vi "Create New Tags and Mappings.vi"(8 "write reservations in":cluster{"Array":T1[]}[](array[cluster]), 9 "read reservations in":cluster{"Array":T1[]}[](array[cluster]), 10 "module mapping":T2[](array[typedef]), 11 "main data dictionary in":refnum<class "data dictionary.lvclass">) -> (2 "module mapping":T2[](array[typedef]), 3 "main data dictionary out":refnum<class "data dictionary.lvclass">)   [LabVIEW 2013, in "Engine Runtime Interface.lvclass"]
uses:
  Engine Runtime Interface.lvclass
  Engine Configuration/Module Mappings.ctl
  <vilib>/NI/Tag Bus/table/mapping specification.ctl
  <vilib>/NI/Tag Bus/tag/Data Type.ctl
  <vilib>/NI/Tag Bus/table/mapping.ctl
  <vilib>/NI/Tag Bus/dictionary/data dictionary.lvclass
  <vilib>/NI/Tag Bus Module Framework/module configuration/channel reservation.ctl
  <vilib>/NI/Tag Bus Module Framework/channel/TBM channel.lvclass
  <vilib>/NI/Tag Bus/tag/tag descriptor.lvclass
  Engine Configuration/engine configuration.lvclass
  <vilib>/NI/Tag Bus/table/data table.lvlib
  <vilib>/NI/Tag Bus Module Framework/module configuration/TBM module configuration.lvclass
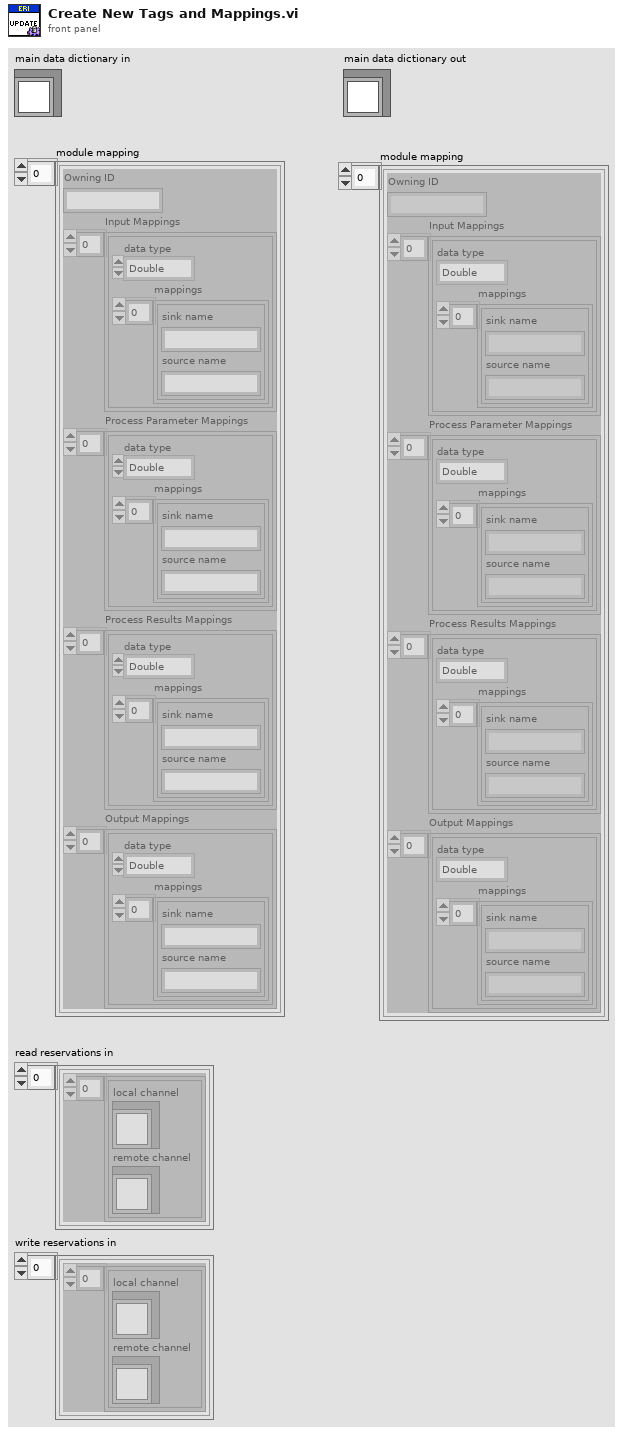
[diagram p1: front panel]
types:
  T1 = typedef "TBM module configuration.lvclass/channel reservation.ctl" = cluster{"local channel":refnum<class "TBM channel.lvclass">, "remote channel":refnum<class "TBM channel.lvclass">}
  T2 = typedef "engine configuration.lvclass/Module Mappings.ctl" = cluster{"Owning ID":string, "Input Mappings":T3[], "Process Parameter Mappings":T3[], "Process Results Mappings":T3[], "Output Mappings":T3[]}
  T3 = typedef "tag bus.lvlib/data table.lvlib/mapping specification.ctl" = cluster{"data type":T4, "mappings":T5[]}
  T4 = typedef "tag bus.lvlib/tag descriptor.lvclass/Data Type.ctl" = enum16{"Double", "Single", "I64", "I32", "I16", "I8", "U64", "U32", "U16", "U8", "Boolean", "String", "Array of Double", "Array of Single", "Array of I64", "Array of I32", "Array of I16", "Array of I8", "Array of U64", "Array of U32", "Array of U16", "Array of U8", "Array of Boolean", "Array of String"}
  T5 = typedef "tag bus.lvlib/data table.lvlib/mapping.ctl" = cluster{"sink name":string, "source name":string}
  T6 = cluster{"Tag Name":string, "Channel Name":string}
  T7 = cluster{"Tag Name":string, "Channel Name":string}[]
  T8 = typedef "engine configuration.lvclass/Mappings.ctl" = cluster{"Data Type":T4, "Mappings":cluster{"Tag Name":string, "Channel Name":string}[]}
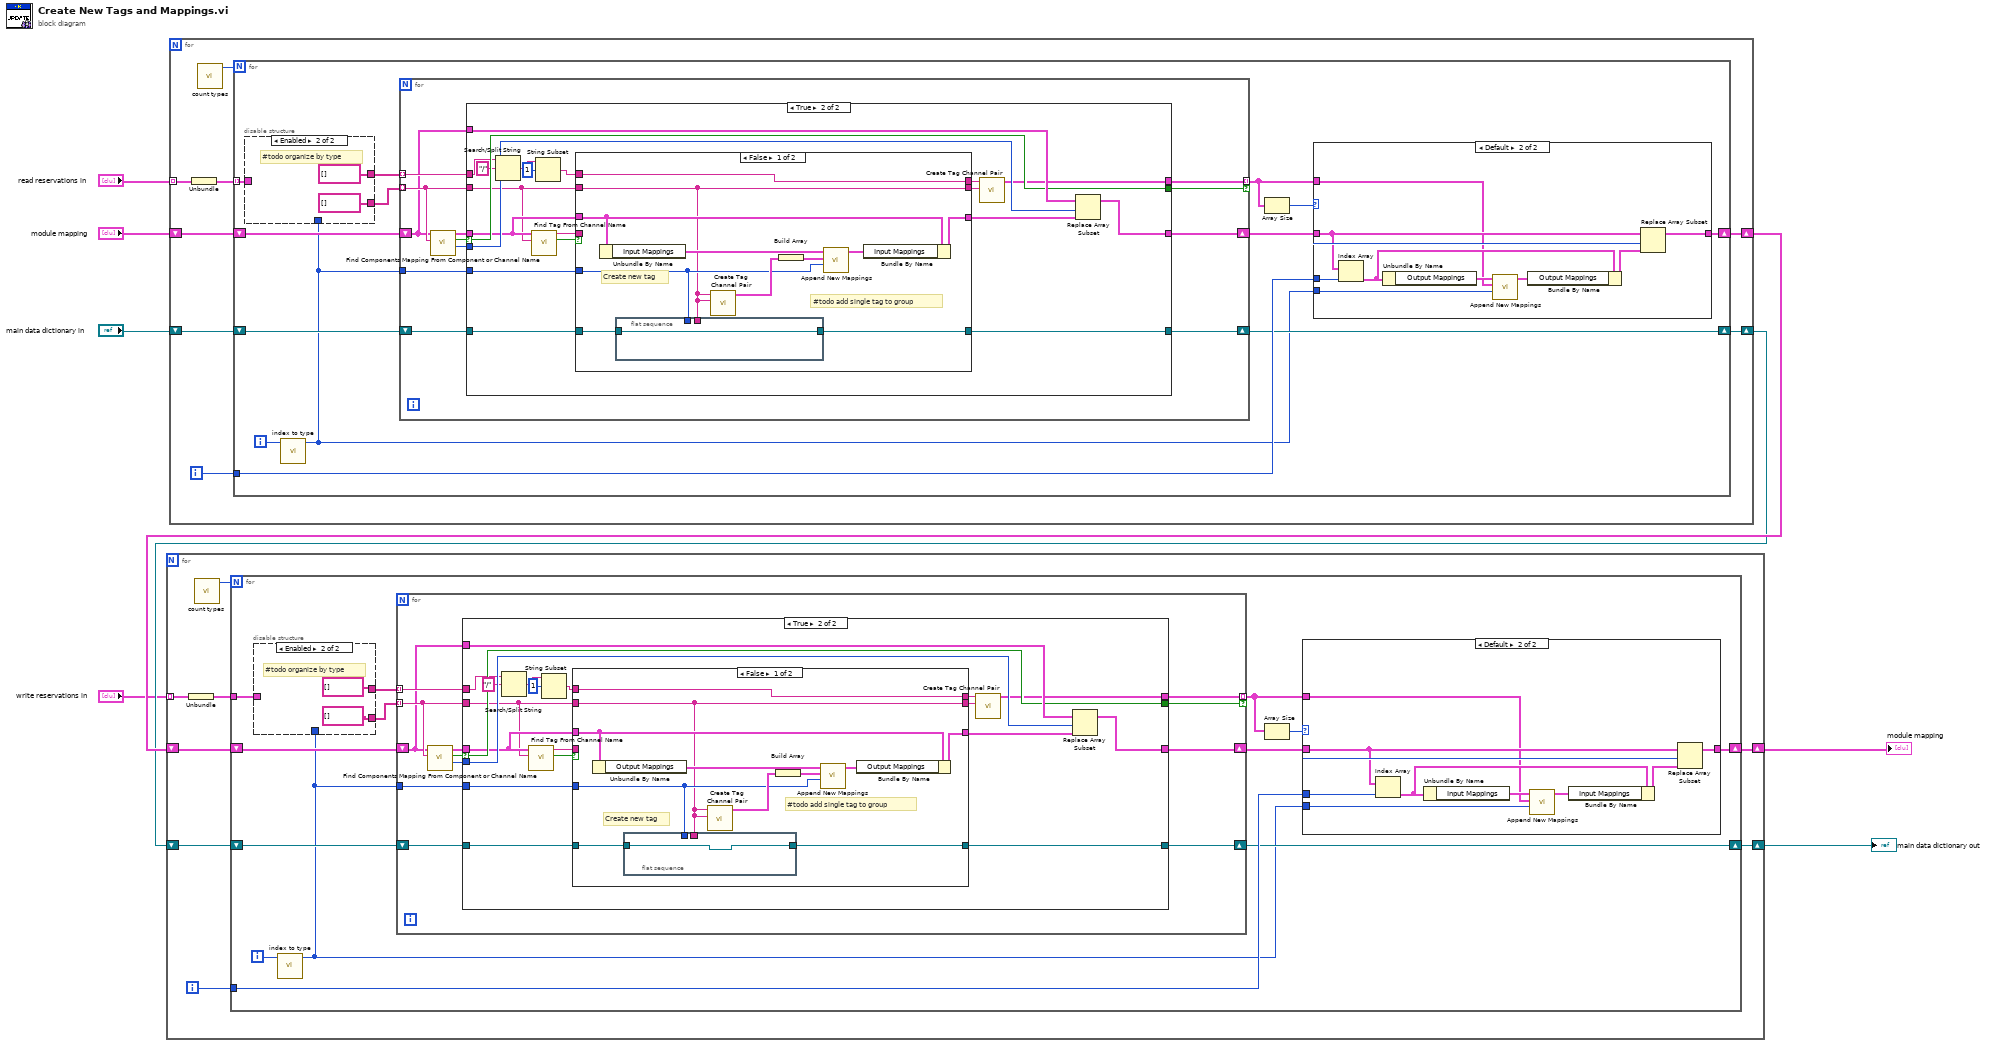
[diagram p0: block diagram]
diagram:
  n1 = for {
    tunnel: "read reservations in" -> [w16] mode=indexing
    shift-right: [w15] -> w6
    shift-left: "module mapping" -> [w12]
    shift-right: [w13] -> w5
    shift-left: "main data dictionary in" -> [w11]
    i -> [w14]
    n2 = Unbundle(w16) -> ("Array"=w9:T1[])
    n3 = call <vilib>:"count types.vi"() -> ("type count"=w10:i32)  [unwired: 11 in]
    n4 = for {
      N: w10 -> [_]
      tunnel: w9 -> [w22] mode=indexing
      tunnel: w14 -> [w28]
      shift-right: [w29] -> w15
      shift-left: w12 -> [w26]
      shift-right: [w27] -> w13
      shift-left: w11 -> [w25]
      i -> [w24]
      n5 = call <vilib>:"index to type.vi"("I32"=w24) -> ("type"=w19:T4)  [unwired: 10 in]
      n6 = disable-structure shown="Enabled" {
        disable-tunnel: w22 -> [_ _]
        disable-tunnel: [_ string[] [] ("tags")] -> w21
        disable-tunnel: [_ string[] [] ("tags")] -> w20
        disable-tunnel: w19 -> [_ _]
        frame Disabled {
        }
        frame Enabled {
          # "#todo organize by type"
        }
      }
      n7 = for {
        tunnel: w20 -> [w53] mode=indexing
        tunnel: [w52] -> w18 mode=indexing if=w44
        tunnel: w21 -> [w50] mode=indexing
        shift-right: [w46] -> w23
        shift-left: w26 -> [w47]
        shift-right: [w43] -> w27
        shift-left: w25 -> [w51]
        tunnel: w19 -> [w42]
        n8 = call "Find Components Mapping From Component or Channel Name.vi"("module/channel name"=w50, "module mapping"=w47) -> ("index"=w48:i32, "found?"=w45:bool, "found mapping"=w49:T2)  [unwired: 7 in]
        n9 = case shown="True" w45 {
          selector: w45 -> [w55 w71]
          tunnel: w53 -> [_ w61]
          tunnel: [_ w65] -> w52
          tunnel: w51 -> [w54 w76]
          tunnel: w50 -> [_ w68]
          tunnel: w49 -> [_ w69]
          tunnel: w48 -> [_ w74]
          tunnel: w47 -> [w56 w73]
          tunnel: [w56 w72] -> w46
          tunnel: [w55 w71] -> w44
          tunnel: [w54 w70] -> w43
          tunnel: w42 -> [_ w62]
          frame False {
          }
          frame True {
            n10 = Search/Split String(string=w61, search string/char (-)="/") -> (match + rest of string=w59:string)  [unwired: 1 in, 2 out]
            n11 = call "Find Tag From Channel Name.vi"("channel name"=w68, "Module Mappings"=w69) -> ("found?"=w67:bool, "mapped tag"=w66:string)  [unwired: 8 in]
            n12 = String Subset(string=w59, offset (0)=1) -> (substring=w57:string)  [unwired: 1 in]
            n13 = case shown="False" w67 {
              tunnel: w57 -> [w81 w90]
              tunnel: w66 -> [_ w89]
              tunnel: w68 -> [w77 _]
              tunnel: w76 -> [w80 w91]
              tunnel: w69 -> [w87 w92]
              tunnel: [w86 w92] -> w75
              tunnel: [w79 w91] -> w70
              tunnel: [w81 w90] -> w64
              tunnel: [w77 w89] -> w63
              tunnel: w62 -> [w78 _]
              frame False {
                # "#todo add single tag to group"
                # "Create new tag"
                n14 = Unbundle By Name(w87) -> ("Input Mappings"=w85:T3[])
                n15 = flat-sequence {
                  tunnel: w80 -> [w88]
                  tunnel: [w88] -> w79
                  tunnel: w78 -> [_]
                  tunnel: w77 -> [_]
                  frame #0 {
                  }
                }
                n16 = call "Create Tag Channel Pair.vi"("Tag Name"=w77, "Channel Name"=w77) -> ("tag channel pair"=w83:T6)  [unwired: 9 in]
                n17 = Build Array(w83) -> (w82:T7)
                n18 = call "Append New Mappings.vi"("Type"=w78, "Mappings to Append"=w82, "Mappings in"=w85) -> ("Mappings out"=w84:T8[])  [unwired: 8 in]
                n19 = Bundle By Name(cluster=w87, "Input Mappings"=w84) -> (w86:T2)
              }
              frame True {
              }
            }
            n20 = call "Create Tag Channel Pair.vi"("Tag Name"=w63, "Channel Name"=w64) -> ("tag channel pair"=w65:T6)  [unwired: 9 in]
            n21 = Replace Array Subset(array=w73, new element=w75, index=w74) -> (w72:T2[])
          }
        }
      }
      n22 = Array Size(array=w18) -> (size(s)=w17:i32)
      n23 = case shown="Default" w17 {
        tunnel: [w32 w41] -> w29
        tunnel: w28 -> [_ w40]
        tunnel: w23 -> [w32 w36]
        tunnel: w19 -> [_ w34]
        tunnel: w18 -> [_ w33]
        frame 0 {
        }
        frame Default {
          n24 = Index Array(array=w36, index=w40) -> (element=w39:T2)
          n25 = Unbundle By Name(w39) -> ("Output Mappings"=w35:T3[])
          n26 = call "Append New Mappings.vi"("Type"=w34, "Mappings to Append"=w33, "Mappings in"=w35) -> ("Mappings out"=w38:T8[])  [unwired: 8 in]
          n27 = Bundle By Name(cluster=w39, "Output Mappings"=w38) -> (w37:T2)
          n28 = Replace Array Subset(array=w36, new element=w37, index=w40) -> (w41:T2[])
        }
      }
    }
  }
  n29 = for {
    tunnel: "write reservations in" -> [w100] mode=indexing
    shift-right: [w99] -> w7
    shift-left: w6 -> [w96]
    shift-right: [w97] -> w3
    shift-left: w5 -> [w95]
    i -> [w98]
    n30 = Unbundle(w100) -> ("Array"=w93:T1[])
    n31 = call <vilib>:"count types.vi"() -> ("type count"=w94:i32)  [unwired: 11 in]
    n32 = for {
      N: w94 -> [_]
      tunnel: w93 -> [w106]
      tunnel: w98 -> [w112]
      shift-right: [w113] -> w99
      shift-left: w96 -> [w110]
      shift-right: [w111] -> w97
      shift-left: w95 -> [w109]
      i -> [w108]
      n33 = call <vilib>:"index to type.vi"("I32"=w108) -> ("type"=w103:T4)  [unwired: 10 in]
      n34 = disable-structure shown="Enabled" {
        disable-tunnel: w106 -> [_ _]
        disable-tunnel: [_ string[] [] ("tags")] -> w105
        disable-tunnel: [_ string[] [] ("tags")] -> w104
        disable-tunnel: w103 -> [_ _]
        frame Disabled {
        }
        frame Enabled {
          # "#todo organize by type"
        }
      }
      n35 = for {
        tunnel: w104 -> [w137] mode=indexing
        tunnel: [w136] -> w102 mode=indexing if=w128
        tunnel: w105 -> [w134] mode=indexing
        shift-right: [w130] -> w107
        shift-left: w110 -> [w131]
        shift-right: [w127] -> w111
        shift-left: w109 -> [w135]
        tunnel: w103 -> [w126]
        n36 = call "Find Components Mapping From Component or Channel Name.vi"("module/channel name"=w134, "module mapping"=w131) -> ("index"=w132:i32, "found?"=w129:bool, "found mapping"=w133:T2)  [unwired: 7 in]
        n37 = case shown="True" w129 {
          selector: w129 -> [w139 w155]
          tunnel: w137 -> [_ w142]
          tunnel: [_ w149] -> w136
          tunnel: w135 -> [w138 w160]
          tunnel: w134 -> [_ w152]
          tunnel: w133 -> [_ w153]
          tunnel: w132 -> [_ w158]
          tunnel: w131 -> [w140 w157]
          tunnel: [w140 w156] -> w130
          tunnel: [w139 w155] -> w128
          tunnel: [w138 w154] -> w127
          tunnel: w126 -> [_ w146]
          frame False {
          }
          frame True {
            n38 = Search/Split String(string=w142, search string/char (-)="/") -> (match + rest of string=w144:string)  [unwired: 1 in, 2 out]
            n39 = call "Find Tag From Channel Name.vi"("channel name"=w152, "Module Mappings"=w153) -> ("found?"=w151:bool, "mapped tag"=w150:string)  [unwired: 8 in]
            n40 = String Subset(string=w144, offset (0)=1) -> (substring=w141:string)  [unwired: 1 in]
            n41 = case shown="False" w151 {
              tunnel: w141 -> [w165 w174]
              tunnel: w150 -> [_ w173]
              tunnel: w152 -> [w161 _]
              tunnel: w160 -> [w164 w175]
              tunnel: w153 -> [w171 w176]
              tunnel: [w170 w176] -> w159
              tunnel: [w163 w175] -> w154
              tunnel: [w165 w174] -> w148
              tunnel: [w161 w173] -> w147
              tunnel: w146 -> [w162 _]
              frame False {
                # "#todo add single tag to group"
                # "Create new tag"
                n42 = Unbundle By Name(w171) -> ("Output Mappings"=w169:T3[])
                n43 = flat-sequence {
                  tunnel: w164 -> [w172]
                  tunnel: [w172] -> w163
                  tunnel: w162 -> [_]
                  tunnel: w161 -> [_]
                  frame #0 {
                  }
                }
                n44 = call "Create Tag Channel Pair.vi"("Tag Name"=w161, "Channel Name"=w161) -> ("tag channel pair"=w167:T6)  [unwired: 9 in]
                n45 = Build Array(w167) -> (w166:T7)
                n46 = call "Append New Mappings.vi"("Type"=w162, "Mappings to Append"=w166, "Mappings in"=w169) -> ("Mappings out"=w168:T8[])  [unwired: 8 in]
                n47 = Bundle By Name(cluster=w171, "Output Mappings"=w168) -> (w170:T2)
              }
              frame True {
              }
            }
            n48 = call "Create Tag Channel Pair.vi"("Tag Name"=w147, "Channel Name"=w148) -> ("tag channel pair"=w149:T6)  [unwired: 9 in]
            n49 = Replace Array Subset(array=w157, new element=w159, index=w158) -> (w156:T2[])
          }
        }
      }
      n50 = Array Size(array=w102) -> (size(s)=w101:i32)
      n51 = case shown="Default" w101 {
        tunnel: [w116 w125] -> w113
        tunnel: w112 -> [_ w124]
        tunnel: w107 -> [w116 w120]
        tunnel: w102 -> [_ w118]
        tunnel: w103 -> [_ w117]
        frame 0 {
        }
        frame Default {
          n52 = Index Array(array=w120, index=w124) -> (element=w123:T2)
          n53 = Unbundle By Name(w123) -> ("Input Mappings"=w119:T3[])
          n54 = call "Append New Mappings.vi"("Type"=w117, "Mappings to Append"=w118, "Mappings in"=w119) -> ("Mappings out"=w122:T8[])  [unwired: 8 in]
          n55 = Bundle By Name(cluster=w123, "Input Mappings"=w122) -> (w121:T2)
          n56 = Replace Array Subset(array=w120, new element=w121, index=w124) -> (w125:T2[])
        }
      }
    }
  }
  "module mapping" <- w7
  "main data dictionary out" <- w3
